vi "threhsold IMAQ.vi"(8 "error in (no error)":errorcluster, 9 "Threshold high":dbl, 10 "Threshold":dbl, 11 "Refnum in":T1) -> (0 "error out":errorcluster, 1 "Maximal Value":sgl, 2 "Mean Value":sgl, 3 "Refnum out":T1(plugin-control))   [LabVIEW 2020]
uses:
  IMAQ Image.ctl
  NI_Vision_Development_Module.lvlib
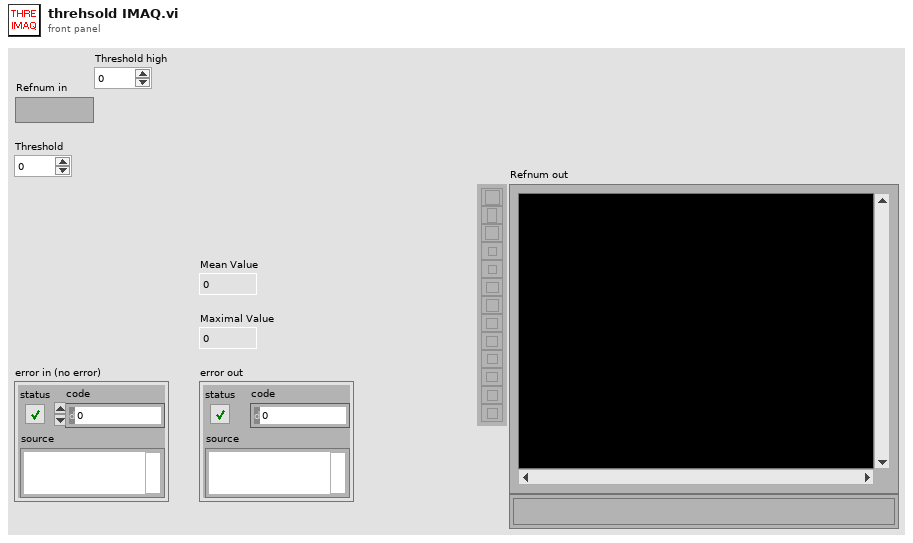
[diagram p1: front panel]
types:
  T1 = typedef "IMAQ Image.ctl" = refnum<image>
  T2 = cluster{"histogram":u32[], "Minimal Value":sgl, "Maximal Value":sgl, "Starting Value":sgl, "Interval Width":sgl, "Mean Value":sgl, "Standard  Variation":sgl, "Area (pixels)":i32}
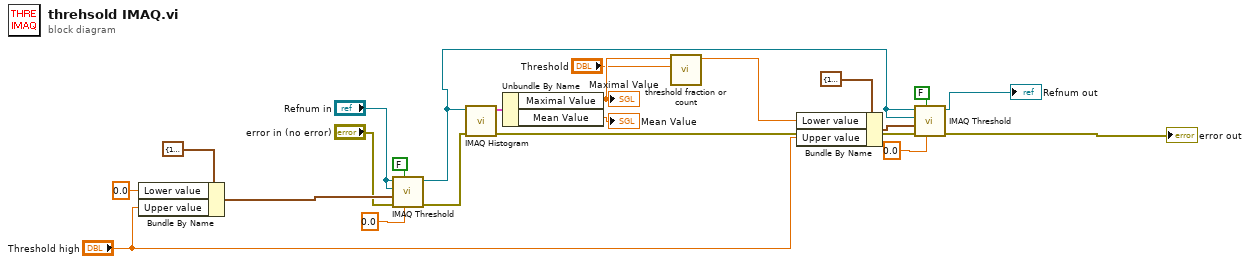
[diagram p0: block diagram]
diagram:
  n1 = Bundle By Name(cluster=cluster{"Lower value":sgl, "Upper value":sgl} {"Lower value"=100.0, "Upper value"=9999999.0} ("Range"), "Lower value"=sgl 0.0, "Upper value"="Threshold high") -> (w4:cluster{"Lower value":sgl, "Upper value":sgl})
  n2 = call "IMAQ Threshold"("Replace Value"=sgl 0.0, "Keep/Replace Value (Replace)"=FALSE, "error in (no error)"="error in (no error)", "Range"=w4, "Image Dst"="Refnum in", "Image Src"="Refnum in") -> ("error out"=w1:errorcluster, "Image Dst Out"=w3:T1)  [unwired: 4 in]
  n3 = call "IMAQ Histogram"("error in (no error)"=w1, "Image"=w3) -> ("error out"=w17:errorcluster, "Histogram Report"=w12:T2)  [unwired: 8 in]
  n4 = Unbundle By Name(w12) -> ("Maximal Value"=w22:sgl, "Mean Value"=→"Mean Value":sgl)
  "Maximal Value" <- w22
  n5 = call "threshold fraction or count.vi"("Threshold in"="Threshold", "Maximal Value"=w22) -> ("Threshold out"=w18:dbl)  [unwired: 9 in]
  n6 = Bundle By Name(cluster=cluster{"Lower value":sgl, "Upper value":sgl} {"Lower value"=100.0, "Upper value"=9999999.0} ("Range"), "Lower value"=w18, "Upper value"="Threshold high") -> (w13:cluster{"Lower value":sgl, "Upper value":sgl})
  n7 = call "IMAQ Threshold"("Replace Value"=sgl 0.0, "Keep/Replace Value (Replace)"=FALSE, "error in (no error)"=w17, "Range"=w13, "Image Dst"=w3, "Image Src"=w3) -> ("error out"=→"error out":errorcluster, "Image Dst Out"=→"Refnum out":T1)  [unwired: 4 in]
